vi "PrecessVirtual.vi"(0 "RA_texto_rad":string="0" caption="Right Ascension", 1 "DEC_texto_rad":string="0" caption="Declination") -> (2 "AZIMUTE":dbl format="%#.6g", 3 "ZENITAL ANGLE":dbl format="%#.6g", 4 "Sideral Time":dbl format="%#.9g", 5 "RA":dbl format="%#.9f", 6 "AH":dbl format="%#.9g", 7 "DEC":dbl format="%#.9g")   [LabVIEW 2012]
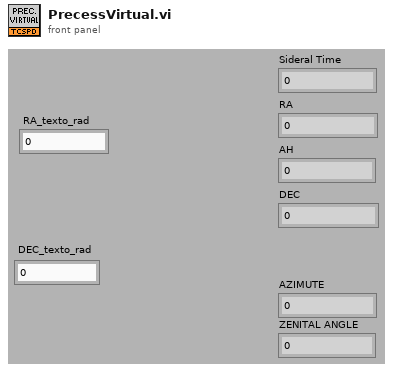
[diagram p1: front panel]
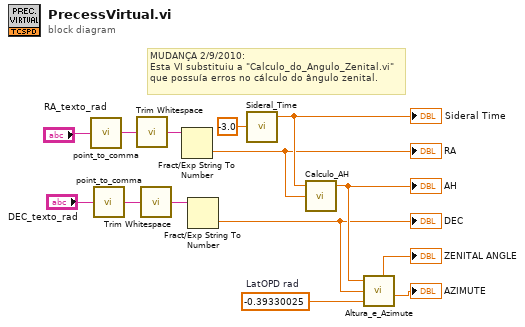
[diagram p0: block diagram]
diagram:
  w1 = -0.39330025  # LatOPD rad
  # "MUDANÇA 2/9/2010:\nEsta VI substituiu a \"Calculo_do_Angulo_Zenital.vi\" que possuía erros no cálculo do ângulo zenital."
  n1 = call "point_to_comma.vi"("Lat_A"="RA_texto_rad") -> ("Saída"=w12:string)
  n2 = call "point_to_comma.vi"("Lat_A"="DEC_texto_rad") -> ("Saída"=w11:string)
  n3 = call <vilib>:"Trim Whitespace.vi"("string"=w12) -> ("trimmed string"=w6:string)  [unwired: 1 in]
  n4 = call <vilib>:"Trim Whitespace.vi"("string"=w11) -> ("trimmed string"=w7:string)  [unwired: 1 in]
  n5 = Fract/Exp String To Number(string=w6) -> (number=w9:dbl)  [unwired: 3 in, 1 out]
  "RA" <- w9
  n6 = Fract/Exp String To Number(string=w7) -> (number=w2:dbl)  [unwired: 3 in, 1 out]
  "DEC" <- w2
  n7 = call "Sideral_Time.vi"("Fuso"=-3.0) -> ("Sideral Time"=w14:dbl)  [unwired: 2 in, 2 out]
  "Sideral Time" <- w14
  n8 = call "Calculo_AH.vi"("RA_Destino"=w9, "Hora Sideral"=w14) -> ("AH_Destino"=w3:dbl)  [unwired: 1 in, 2 out]
  "AH" <- w3
  n9 = call "Altura_e_Azimute.vi"("LAT rad"=w1, "DEC rad"=w2, "AH rad"=w3) -> ("AZIMUTE rad"=→"AZIMUTE":dbl, "ANG. ZENITAL rad"=→"ZENITAL ANGLE":dbl)  [unwired: 4 out]
